vi "FilesAndOutputPathMap.vi"() -> ()   [LabVIEW 2017]
uses:
  JsonConverters/SourceJsonPaths.ctl
panel:
  in  "Files and output map":T1[](array[typedef])
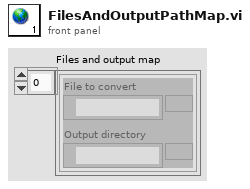
[diagram p1: front panel]
types:
  T1 = typedef "SourceJsonPaths.ctl" = cluster{"File to convert":path, "Output directory":path}
diagram:
